vi "Comma List to String Array.vi"(11 "String":string) -> (3 "Array":string[](array[string]))   [LabVIEW 2011]
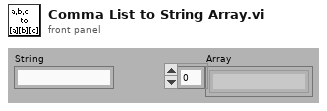
[diagram p1: front panel]
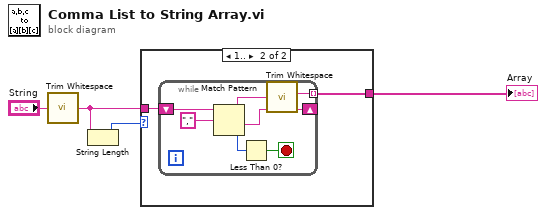
[diagram p0: block diagram]
diagram:
  n1 = call <vilib>:"Trim Whitespace.vi"("string"="String") -> ("trimmed string"=w2:string)  [unwired: 1 in]
  n2 = String Length(string=w2) -> (length=w1:i32)
  n3 = case shown="1.." w1 {
    tunnel: [_ w6] -> w4
    tunnel: w2 -> [_ w5]
    frame Default {
      # "no elements"
    }
    frame 1.. {
      n4 = while {
        shift-right: [w9] -> _
        shift-left: w5 -> [w13]
        tunnel: [w7] -> w6 mode=indexing
        stop <- w11 stop-if-true
        n5 = Match Pattern(string=w13, regular expression=",") -> (before substring=w8:string, after substring=w9:string, offset past match=w10:i32)  [unwired: 2 out]
        n6 = Less Than 0?(x=w10) -> (x < 0?=w11:bool)
        n7 = call <vilib>:"Trim Whitespace.vi"("string"=w8) -> ("trimmed string"=w7:string)  [unwired: 1 in]
      }
    }
  }
  "Array" <- w4
